vi "LIN USD Request.vi"(5 "Len":u16, 6 "pCmd":string, 7 "NAD":u8, 8 "error in (no error)":errorcluster, 9 "ID":u8, 10 "LINIndex":i32, 11 "DevHandle":i32) -> (0 "error out":errorcluster, 3 "function return":i32, 4 "pCmd out":string)   [LabVIEW 2010, in "usb2lin_ex.lvlib"]
doc: "int WINAPI LIN_USD_Request(int DevHandle,int LINIndex,unsigned char ID,unsigned char NAD,unsigned char *pCmd,unsigned short Len);"
uses:
  usb2lin_ex.lvlib
  USB2XXX.dll
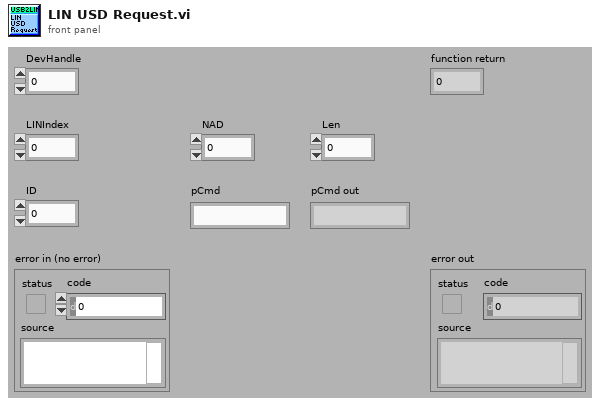
[diagram p1: front panel]
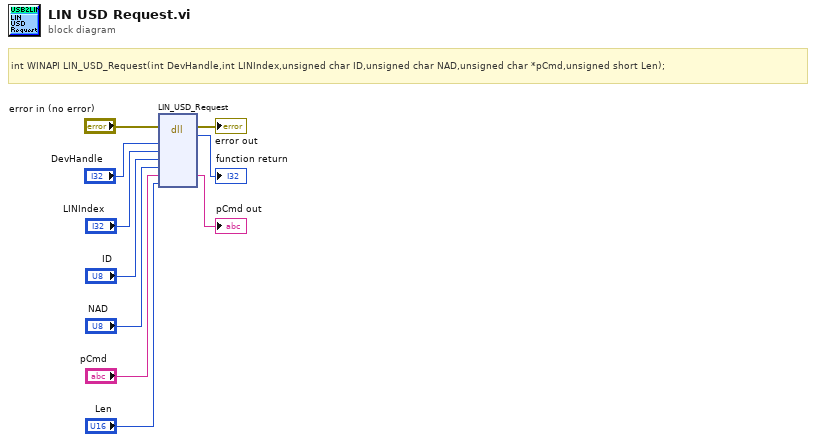
[diagram p0: block diagram]
diagram:
  # "int WINAPI LIN_USD_Request(int DevHandle,int LINIndex,unsigned char ID,unsigned char NAD,unsigned char *pCmd,unsigned short Len);"
  n1 = dll-call lib="E:/OtherWork/STM32/USB2XXX_Example/sdk/api/Labview/USB2XXX.*" fn="LIN_USD_Request"(error in="error in (no error)", "DevHandle"="DevHandle", "LINIndex"="LINIndex", "ID"="ID", "NAD"="NAD", "pCmd"="pCmd", "Len"="Len") -> (error out=→"error out":errorcluster, →"function return":i32, "pCmd"=→"pCmd out":string)  [unwired: 7 in, 1 out]
